vi "ReadUSB.vi"() -> ()   [LabVIEW 2017]
uses:
  <vilib>/Instr/_visa.llb/VISA Configure Serial Port (Instr).vi
panel:
  in  "End":bool
  in  "fc corte 2":dbl=5.0
  out "fps":dbl
  in  "fc corte":dbl=5.0
  out "appended array 2":i32[](array[numeric])
  out "appended array":string[](array[string])
  out "dutycicle":cluster{dbl}(graph)
  out "PWM":dbl
  out "String Tratada 2":string
  out "Aceleração Z":dbl
  out "String Lida":string
  out "config error":errorcluster
  out "String Tratada":string
  out "Gravidade":cluster{dbl}(graph)
  in  "VISA resource name":refnum<visa-resource-name>
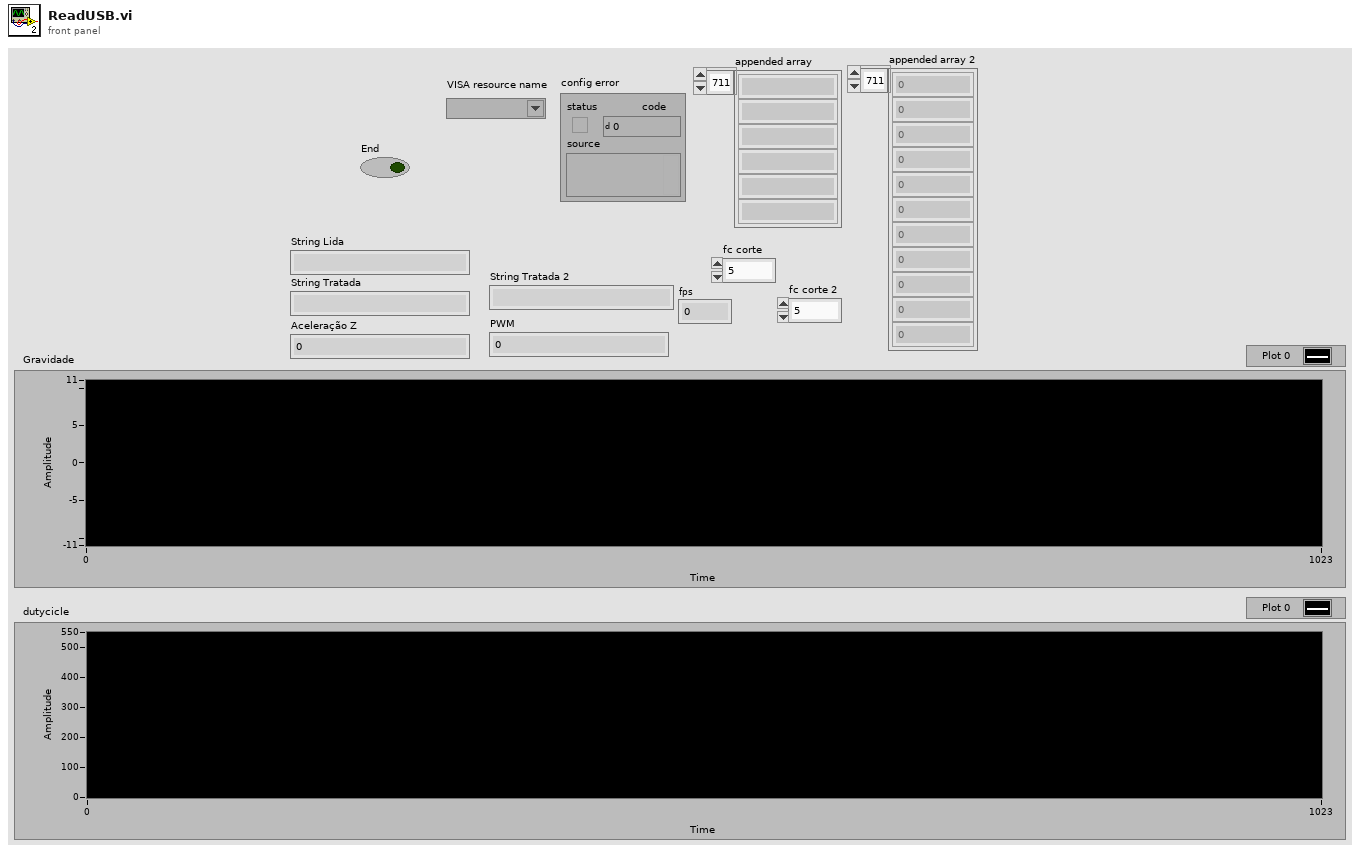
[diagram p1: front panel]
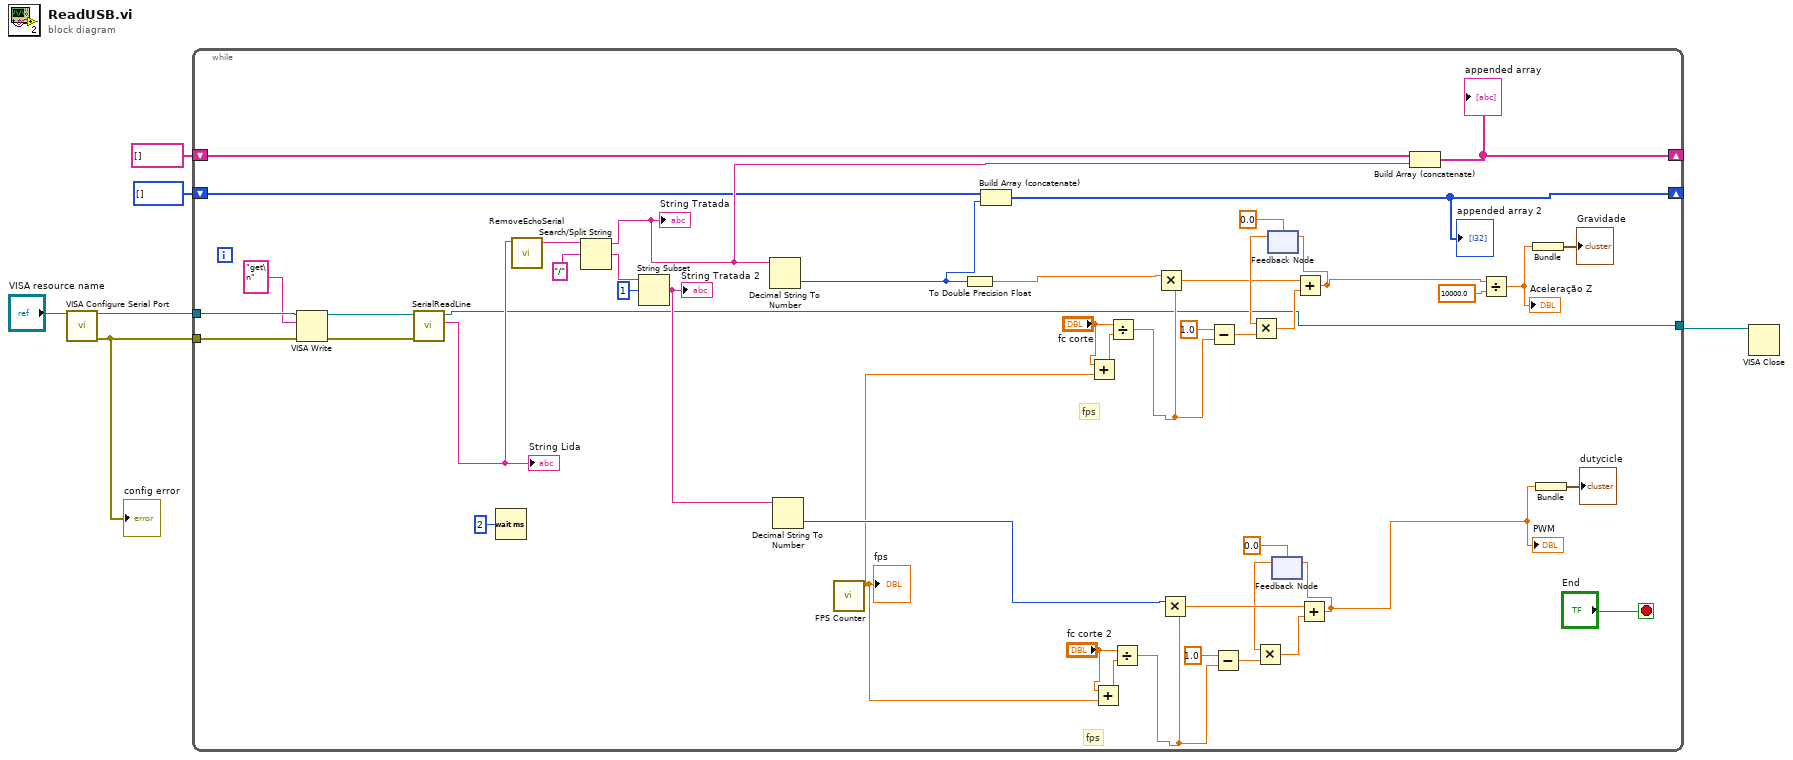
[diagram p0: block diagram]
diagram:
  n1 = call-poly "VISA Configure Serial Port"("VISA resource name"="VISA resource name") -> ("VISA resource name out"=w5:refnum<visa-resource-name>, "error out"=w4:errorcluster)  [unwired: 13 in]
  "config error" <- w4
  n2 = while {
    tunnel: w5 -> [w53]
    tunnel: w4 -> [w52]
    shift-right: [w38] -> _
    shift-left: string[] [] -> [w37]
    shift-right: [w33] -> _
    shift-left: i32[] [] -> [w34]
    tunnel: [w7] -> w1
    stop <- "End" stop-if-true
    # "fps"
    # "fps"
    n3 = VISA Write(VISA resource name=w53, write buffer="get\n", error in (no error)=w52) -> (VISA resource name out=w49:refnum<visa-resource-name>, error out=w48:errorcluster)  [unwired: 1 out]
    n4 = call "SerialReadLine.vi"("error in"=w48, "VISA resource name in"=w49) -> ("String"=w44:string, "VISA resource name out"=w7:refnum<visa-resource-name>)  [unwired: 7 in, 1 out]
    "String Lida" <- w44
    n5 = Wait (ms)(milliseconds to wait=u32 2) -> ()  [unwired: 1 out]
    n6 = call "RemoveEchoSerial.vi"("String in"=w44) -> ("String out"=w36:string)  [unwired: 10 in]
    n7 = Search/Split String(string=w36, search string/char (-)="/") -> (substring before match=w35:string, match + rest of string=w42:string)  [unwired: 1 in, 1 out]
    "String Tratada" <- w35
    n8 = String Subset(string=w42, offset (0)=1) -> (substring=w39:string)  [unwired: 1 in]
    "String Tratada 2" <- w39
    n9 = Decimal String To Number(string=w35) -> (number=w32:i32)  [unwired: 2 in, 1 out]
    n10 = Decimal String To Number(string=w39) -> (number=w10:i32)  [unwired: 2 in, 1 out]
    n11 = call "FPS Counter.vi"() -> ("Numeric"=w8:dbl)  [unwired: 11 in]
    "fps" <- w8
    n12 = To Double Precision Float(number=w32) -> (double precision float=w21:dbl)
    n13 = Build Array (concatenate)(w34, w32) -> (w33:i32[])
    "appended array 2" <- w33
    n14 = Add(x="fc corte", y=w8) -> (x+y=w24:dbl)
    n15 = Add(x="fc corte 2", y=w8) -> (x+y=w17:dbl)
    n16 = Divide(x="fc corte", y=w24) -> (x/y=w22:dbl)
    n17 = Divide(x="fc corte 2", y=w17) -> (x/y=w19:dbl)
    n18 = Multiply(x=w21, y=w22) -> (x*y=w25:dbl)
    n19 = Multiply(x=w10, y=w19) -> (x*y=w16:dbl)
    n20 = Subtract(x=1.0, y=w22) -> (x-y=w27:dbl)
    n21 = Subtract(x=1.0, y=w19) -> (x-y=w14:dbl)
    n22 = feedback #1(0.0) -> (w28:dbl)
    n23 = Multiply(x=w28, y=w27) -> (x*y=w29:dbl)
    n24 = feedback #2(0.0) -> (w13:dbl)
    n25 = Multiply(x=w13, y=w14) -> (x*y=w12:dbl)
    n26 = Add(x=w25, y=w29) -> (x+y=w20:dbl)
    n27 = feedback-in #1(w20) -> ()
    n28 = Add(x=w16, y=w12) -> (x+y=w9:dbl)
    "PWM" <- w9
    n29 = feedback-in #2(w9) -> ()
    n30 = Build Array (concatenate)(w37, w35) -> (w38:string[])
    "appended array" <- w38
    n31 = Divide(x=w20, y=10000.0) -> (x/y=w45:dbl)
    "Aceleração Z" <- w45
    n32 = Bundle(w45) -> (→"Gravidade":cluster{dbl})  [unwired: 1 in]
    n33 = Bundle(w9) -> (→"dutycicle":cluster{dbl})  [unwired: 1 in]
  }
  n34 = VISA Close(VISA resource name=w1) -> ()  [unwired: 1 in, 1 out]
